vi "Test_ADD_BIN.vi"() -> ()   [LabVIEW 2022 SP3]
panel:
  out "SUM":i16
  in  "Array":bool[](array[boolean])
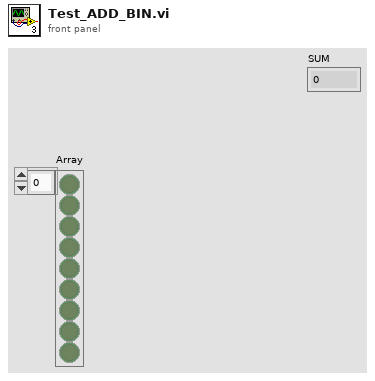
[diagram p1: front panel]
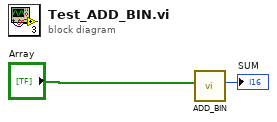
[diagram p0: block diagram]
diagram:
  n1 = call "ADD_BIN.vi"("Array"="Array") -> ("SUM"=→"SUM":i16)  [unwired: 10 in]
